vi "get_radius.vi"(8 "error in (no error)":errorcluster, 11 "TrajectoryDL110420DoubleCircle in":refnum<class "TrajectoryDL110420DoubleCircle.lvclass">) -> (0 "error out":errorcluster, 2 "radius":dbl[unit], 3 "TrajectoryDL110420DoubleCircle out":refnum<class "TrajectoryDL110420DoubleCircle.lvclass">)   [LabVIEW 2010, in "TrajectoryDL110420DoubleCircle.lvclass"]
uses:
  TrajectoryDL110420DoubleCircle.lvclass
  common/classes/SpaceVector/SpaceVector/SpaceVector.lvclass
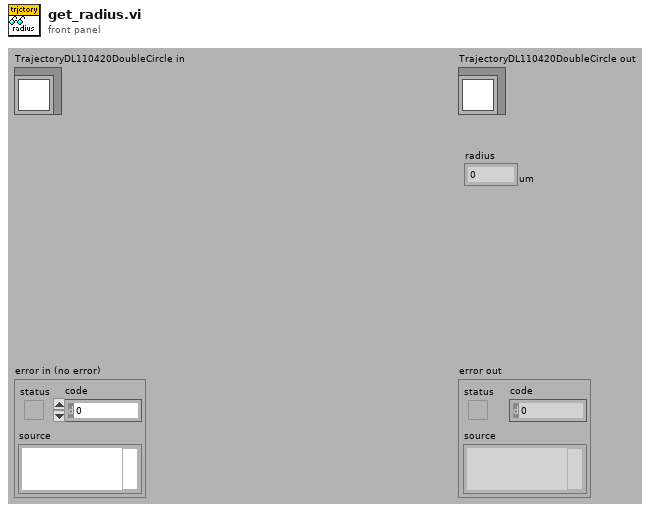
[diagram p1: front panel]
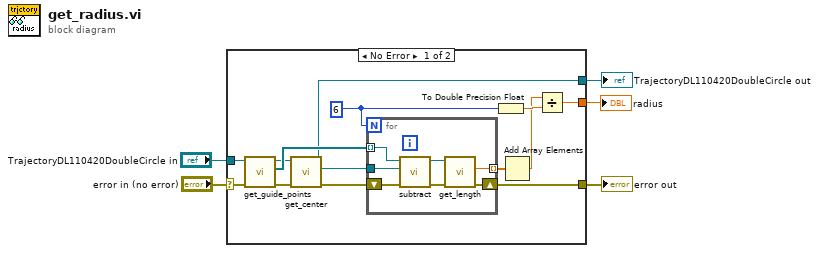
[diagram p0: block diagram]
diagram:
  n1 = case shown="No Error" "error in (no error)" {
    selector: "error in (no error)" -> [w11 w28]
    tunnel: [w16 w28] -> w4
    tunnel: [w6 w27] -> w2
    tunnel: "TrajectoryDL110420DoubleCircle in" -> [w9 w27]
    tunnel: [w15 _] -> w1
    frame No Error {
      w14 = 6 ("number")
      n2 = call-dynamic "get_guide_points.vi"("error in (no error)"=w11, "TrajectoryDL110420DoubleCircle in"=w9) -> ("error out"=w10:errorcluster, "guide points"=w8:refnum<class "SpaceVector.lvclass">[], "TrajectoryDL110420DoubleCircle out"=w7:refnum<class "TrajectoryDL110420DoubleCircle.lvclass">)  [unwired: 7 in]
      n3 = call-dynamic "get_center.vi"("error in (no error)"=w10, "TrajectoryDL110420DoubleCircle in"=w7) -> ("error out"=w13:errorcluster, "center"=w12:refnum<class "SpaceVector.lvclass">, "TrajectoryDL110420DoubleCircle out"=w6:refnum<class "TrajectoryDL110420DoubleCircle.lvclass">)  [unwired: 7 in]
      n4 = for {
        N: w14 -> [_]
        tunnel: w8 -> [w25] mode=indexing
        tunnel: w12 -> [w24]
        shift-right: [w22] -> w16
        shift-left: w13 -> [w26]
        tunnel: [w21] -> w18 mode=indexing
        n5 = call "subtract.vi"("error in (no error)"=w26, "subtrahend"=w24, "SpaceVector in"=w25) -> ("error out"=w23:errorcluster, "SpaceVector out"=w20:refnum<class "SpaceVector.lvclass">)  [unwired: 7 in]
        n6 = call "get_length.vi"("error in (no error)"=w23, "SpaceVector in"=w20) -> ("error out"=w22:errorcluster, "length"=w21:dbl[unit])  [unwired: 7 in, 1 out]
      }
      n7 = To Double Precision Float(number=w14) -> (double precision float=w19:dbl)
      n8 = Add Array Elements(numeric array=w18) -> (sum=w17:dbl[unit])
      n9 = Divide(x=w17, y=w19) -> (x/y=w15:dbl[unit])
    }
    frame Error {
    }
  }
  "error out" <- w4
  "TrajectoryDL110420DoubleCircle out" <- w2
  "radius" <- w1
